vi "WPI_CounterSetMaxPeriod.vi"(8 "error in (no error)":errorcluster, 10 "MaxPeriod (sec)":dbl=0.05, 11 "CounterDevRef in":T1) -> (0 "error out":errorcluster, 3 "CounterDevRef out":T1)   [LabVIEW 2017]
doc: "Specifies the maximum time between pulses that can elapse before the application considers the counter stopped. Use the Get VI to determine whether the counter is stopped.\n\nThis software is licensed. Open the labview\\readme\\WPI Robotics Library Open Source License.txt file for more information."
uses:
  <vilib>/Rock Robotics/WPI/Counter/WPI_CounterDevRef.ctl
  <vilib>/Rock Robotics/SystemInterfaces/Counter/FPGA_CounterCtrSystemIndex.ctl
  <vilib>/Rock Robotics/SystemInterfaces/Counter/FPGA_CounterERRInvalidResource.vi
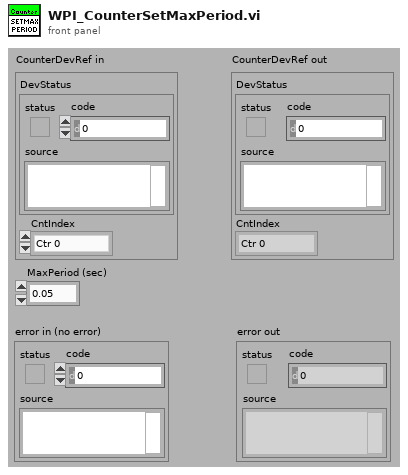
[diagram p1: front panel]
types:
  T1 = typedef "WPI_CounterDevRef.ctl" = cluster{"DevStatus":errorcluster, "CntIndex":T2}
  T2 = typedef "FPGA_CounterCtrSystemIndex.ctl" = enum8{"Ctr 0", "Ctr 1", "Ctr 2", "Ctr 3", "Ctr 4", "Ctr 5", "Ctr 6", "Ctr 7", "Invalid"}
  T3 = typedef "FPGA_CounterCtrDevRef.ctl" = cluster{"DevStatus":errorcluster, "CntIndex":T2}
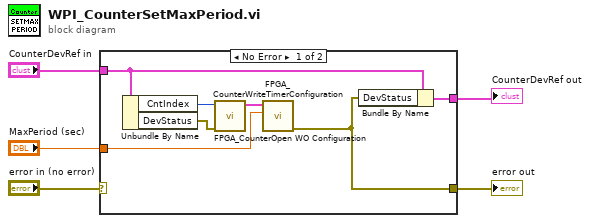
[diagram p0: block diagram]
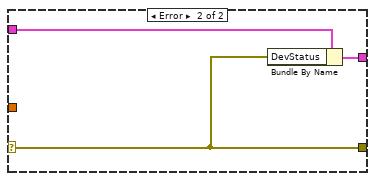
[diagram p2: hidden frame]
diagram:
  n1 = case shown="No Error" "error in (no error)" {
    selector: "error in (no error)" -> [_ w13]
    tunnel: "CounterDevRef in" -> [w12 w15]
    tunnel: [w11 w14] -> w4
    tunnel: [w6 w13] -> w2
    tunnel: "MaxPeriod (sec)" -> [w7 _]
    frame No Error {
      n2 = Unbundle By Name(w12) -> ("CntIndex"=w9:T2, "DevStatus"=w10:errorcluster)
      n3 = call <vilib>:"FPGA_CounterOpen WO Configuration.vi"("error in"=w10, "CntIndex"=w9) -> ("Ctr Ref"=w8:T3)  [unwired: 1 in, 8 out]
      n4 = call <vilib>:"FPGA_CounterWriteTimerConfiguration.vi"("StallPeriod (s)"=w7, "Ctr Ref in"=w8) -> ("error out"=w6:errorcluster)  [unwired: 3 in, 6 out]
      n5 = Bundle By Name(cluster=w12, "DevStatus"=w6) -> (w11:T1)
    }
    frame Error {
      n6 = Bundle By Name(cluster=w15, "DevStatus"=w13) -> (w14:T1)
    }
  }
  "CounterDevRef out" <- w4
  "error out" <- w2
